vi "offTimeCheck.vi"(8 "error in (no error)":errorcluster, 11 "cmd":T1) -> (0 "error out":errorcluster)   [LabVIEW 2019]
uses:
  cmd_offtimecheck.ctl
  _ctrl/rw.ctl
  _ctrl/system-status.ctl
  _ctrl/init-r-stop.ctl
  Durability/common/Global_params.vi
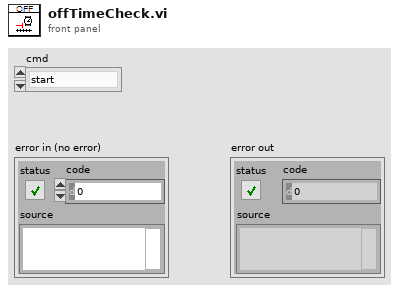
[diagram p1: front panel]
types:
  T1 = typedef "cmd_offtimecheck.ctl" = enum16{"start", "check", "init"}
  T2 = typedef "system-status.ctl" = enum16{"Initial", "Update", "Clear", "Read"}
  T3 = typedef "rw.ctl" = enum16{"read", "write"}
  T4 = typedef "init-r-stop.ctl" = enum16{"ini", "read", "stop"}
  T5 = typedef "cap_config.ctl" = cluster{"Test Mode":enum32{"6.3.2 저온 작동/방치 시험", "6.3.3 고온 작동/방치 시험", "6.3.4 온도 싸이클 시험", "6.3.6 온습도 싸이클 시험", "6.3.8 결로 시험", "6.3.9 빙결 시험"}, "ON time[ms]":dbl, "OFF time[ms]":dbl, "1. 작동시간[분]":dbl, "2. 미작동시간[분]":dbl, "3. 작동시간[분]":dbl, "level[V]":dbl, "duty":dbl, "Freq":dbl, "Voltage+[V]":dbl, "Voltage-[V]":dbl, "Current+[A]":dbl, "Current-[A]":dbl, "출력전압[V]":dbl, "출력전류[A]":dbl, "OVP Level":dbl, "OCP Level":dbl, "Time Div":u16, "Record Len":i32, "방전 기준[V]":dbl, "Repeate (Each Ch)":u32, "Cycle[N]":u32, "ON/OFF 회 수[N]":dbl, "TrigPos[%]":dbl, "시험시간[분]":dbl}
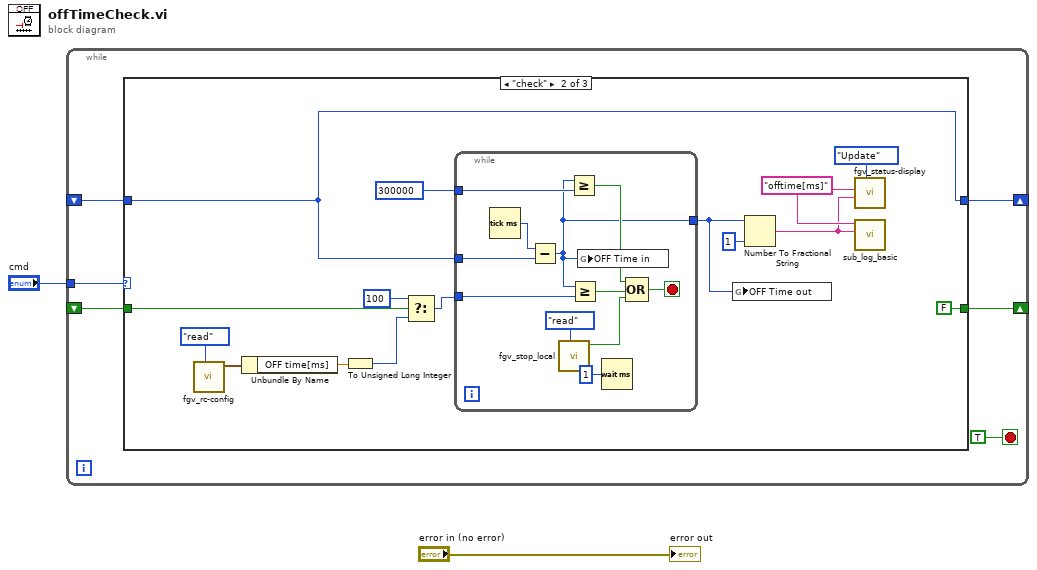
[diagram p0: block diagram]
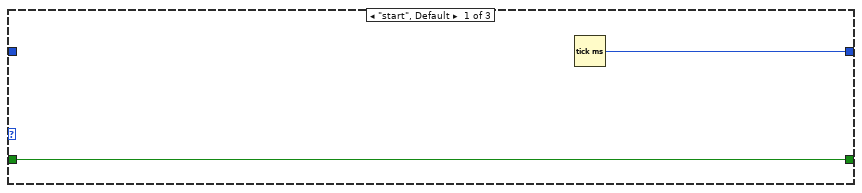
[diagram p2: hidden frame]
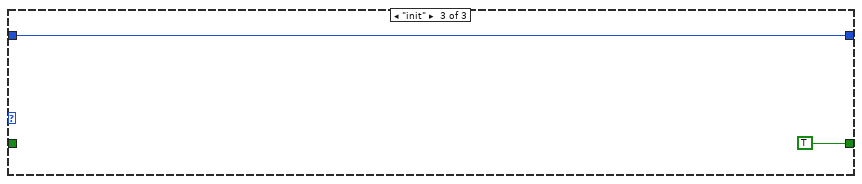
[diagram p3: hidden frame]
diagram:
  n1 = while {
    tunnel: "cmd" -> [w7]
    shift-right: [w6] -> _
    shift-left: _ -> [w5]
    shift-right: [w4] -> _
    shift-left: _ -> [w3]
    stop <- TRUE stop-if-true
    n2 = case shown="\"check\"" w7 {
      tunnel: [w10 w12 w38] -> w6
      tunnel: w5 -> [_ w12 w38]
      tunnel: [w9 FALSE TRUE] -> w4
      tunnel: w3 -> [w9 w16 _]
      frame "start", Default {
        n3 = Tick Count (ms)() -> (millisecond timer value=w10:u32)
      }
      frame "check" {
        w20 = "offtime[ms]" ("title")
        n4 = call "fgv_rc-config.vi"("cmd"=rw."read") -> ("Testconfig out"=w24:T5)  [unwired: 9 in, 1 out]
        n5 = Unbundle By Name(w24) -> ("OFF time[ms]"=w23:dbl)
        n6 = To Unsigned Long Integer(number=w23) -> (unsigned 32bit integer=w15:u32)
        n7 = Select(t=u32 100, s=w16, f=w15) -> (s? t:f=w13:u32)
        n8 = while {
          tunnel: w12 -> [w35]
          tunnel: w13 -> [w34]
          tunnel: u32 300000 ("t1") -> [w32]
          tunnel: [w26] -> w11
          stop <- w27 stop-if-true
          n9 = Tick Count (ms)() -> (millisecond timer value=w36:u32)
          n10 = Subtract(x=w36, y=w35) -> (x-y=w26:u32)
          n11 = call "fgv_stop_local.vi"("cmd"=init-r-stop."read") -> ("stop"=w31:bool)  [unwired: 9 in, 1 out]
          n12 = Greater Or Equal?(x=w26, y=w32) -> (x >= y?=w29:bool)
          n13 = Greater Or Equal?(x=w26, y=w34) -> (x >= y?=w28:bool)
          n14 = global write "Global_params.vi" "OFF Time in"(w26) -> ()
          n15 = Wait (ms)(milliseconds to wait=u32 1) -> ()  [unwired: 1 out]
          n16 = Compound Arithmetic op=OR(w29, w28, w31) -> (w27:bool)
        }
        n17 = global write "Global_params.vi" "OFF Time out"(w11) -> ()
        n18 = Number To Fractional String(number=w11, precision (6)=i16 1) -> (F-format string=w19:string)  [unwired: 2 in]
        n19 = call "fgv_status-display.vi"("Mode"=system-status."Update", "detail"=w19, "title"=w20) -> ()  [unwired: 8 in, 1 out]
        n20 = call "sub_log_basic.vi"("desc"=w19, "Title"=w20) -> ()  [unwired: 9 in, 1 out]
      }
      frame "init" {
      }
    }
  }
  "error out" <- "error in (no error)"
